vi "Read.vi"(8 "error in (no error)":errorcluster, 11 "Boolean in":refnum<class "OnChangeNotifier_CDBL.lvclass">) -> (0 "error out":errorcluster, 2 "Value":T1, 3 "Boolean out":refnum<class "OnChangeNotifier_CDBL.lvclass">)   [LabVIEW 2021, in "OnChangeNotifier_CDBL.lvclass"]
doc: "Abstract Data Classes 2.1.1.13\nTim Streeter - TSA\nCopyright (c) 2025, TSA"
uses:
  OnChangeNotifier_CDBL.lvclass
  Support/Type.ctl
  OnChangeNotifier_CDBL.lvclass/OnChangeNotifier_CDBL.ctl
  <vilib>/TSA/Abstract Data Classes/Abs_Types/Complex Double Float/Abs_Complex Double Float.lvclass
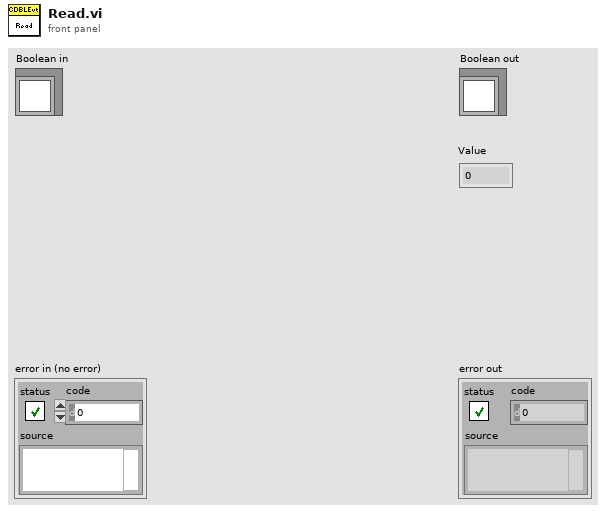
[diagram p1: front panel]
types:
  T1 = typedef "OnChangeNotifier_CDBL.lvclass/Type.ctl" = cdb
  T2 = typedef "OnChangeNotifier_CDBL.lvclass/Class Type.ctl" = refnum<class "Abs_Complex Double Float.lvclass">
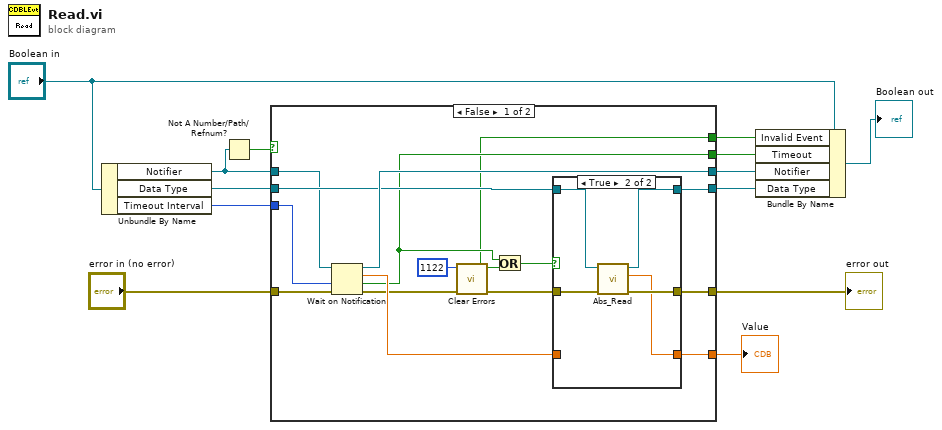
[diagram p0: block diagram]
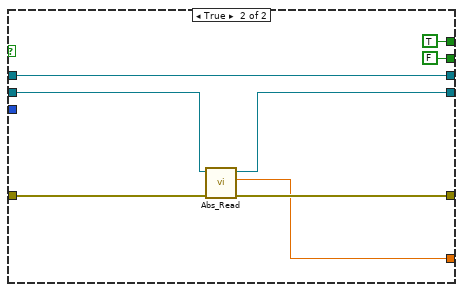
[diagram p3: hidden frame]
diagram:
  n1 = Unbundle By Name("Boolean in") -> ("Notifier"=w2:refnum<notifier>, "Data Type"=w7:T2, "Timeout Interval"=w5:i32)
  n2 = Not A Number/Path/Refnum?(number/path/refnum=w2) -> (NaN/Path/Refnum?=w1:bool)
  n3 = case shown="False" w1 {
    tunnel: [w28 w42] -> w11
    tunnel: "error in (no error)" -> [w27 w44]
    tunnel: [w26 w41] -> w9
    tunnel: [w25 w40] -> w8
    tunnel: w7 -> [w24 w43]
    tunnel: [w23 w39] -> w6
    tunnel: w5 -> [w22 _]
    tunnel: [w19 FALSE ("timed out?")] -> w4
    tunnel: [w17 TRUE ("specific error cleared?")] -> w3
    tunnel: w2 -> [w16 w42]
    frame False {
      n4 = Wait on Notification(notifier=w16, timeout in ms (-1)=w22, error in (no error)=w27) -> (notifier out=w28:refnum<notifier>, notification=w21:T1, timed out?=w19:bool, error out=w14:errorcluster)  [unwired: 1 in]
      n5 = call <vilib>:"Clear Errors.vi"("error in (no error)"=w14, "specific error code to clear (0: all)"=1122) -> ("error out"=w20:errorcluster, "specific error cleared?"=w17:bool)  [unwired: 4 in]
      n6 = Or(x=w19, y=w17) -> (x .or. y?=w18:bool)
      n7 = case shown="True" w18 {
        tunnel: w24 -> [w31 w36]
        tunnel: [w31 w35] -> w26
        tunnel: w20 -> [w30 w34]
        tunnel: [w30 w33] -> w25
        tunnel: [w29 w32] -> w23
        tunnel: w21 -> [w29 _]
        frame False {
        }
        frame True {
          # "Timeout"
          n8 = call-poly <vilib>:"Abs_Read.vi"("error in (no error)"=w34, "Abs_Complex Double Float in"=w36) -> ("error out"=w33:errorcluster, "Value"=w32:cdb, "Abs_Complex Double Float out"=w35:T2)  [unwired: 7 in]
        }
      }
    }
    frame True {
      n9 = call-poly <vilib>:"Abs_Read.vi"("error in (no error)"=w44, "Abs_Complex Double Float in"=w43) -> ("error out"=w40:errorcluster, "Value"=w39:cdb, "Abs_Complex Double Float out"=w41:T2)  [unwired: 7 in]
    }
  }
  "error out" <- w8
  "Value" <- w6
  n10 = Bundle By Name(cluster="Boolean in", "Invalid Event"=w3, "Timeout"=w4, "Notifier"=w11, "Data Type"=w9) -> (→"Boolean out":refnum<class "OnChangeNotifier_CDBL.lvclass">)
